vi "Search 1D Array.vi"(0 "JSON Array":refnum<class "JSON Array.lvclass">, 7 "element":refnum<class "JSON Datatype.lvclass">, 11 "start index (0)":i32) -> (8 "index of element":i32)   [LabVIEW 2017, in "LVJSON.lvlib" / "JSON Array.lvclass"]
uses:
  JSON Array.lvclass
  JSON Datatype/JSON Datatype.lvclass
  JSON Array.lvclass/JSON Array.ctl
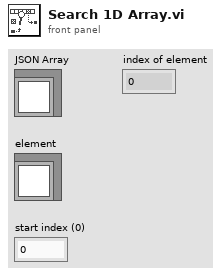
[diagram p1: front panel]
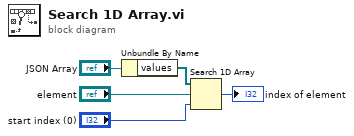
[diagram p0: block diagram]
diagram:
  n1 = Unbundle By Name("JSON Array") -> ("values"=w4:refnum<class "JSON Datatype.lvclass">[])
  n2 = Search 1D Array(1D array=w4, element="element", start index (0)="start index (0)") -> (index of element=→"index of element":i32)
